vi "MosaicFocus.vi"() -> ()   [LabVIEW 2012]
uses:
  <vilib>/Utility/file.llb/Write To Spreadsheet File (DBL).vi
panel:
  in  "Track file":path
  in  "Piezo file":path=path "C:/Users/Ludovico/Lavoro/Experiments/Autofocus/vermi/CONFSTAGELOG/2016_12_16_10_06.txt"
  in  "Stage file":path=path "C:/Users/Ludovico/Lavoro/Experiments/Autofocus/vermi/CONFSTAGELOG/2016_12_16_10_06.txt"
  out "error out":errorcluster
  in  "error in (no error)":errorcluster
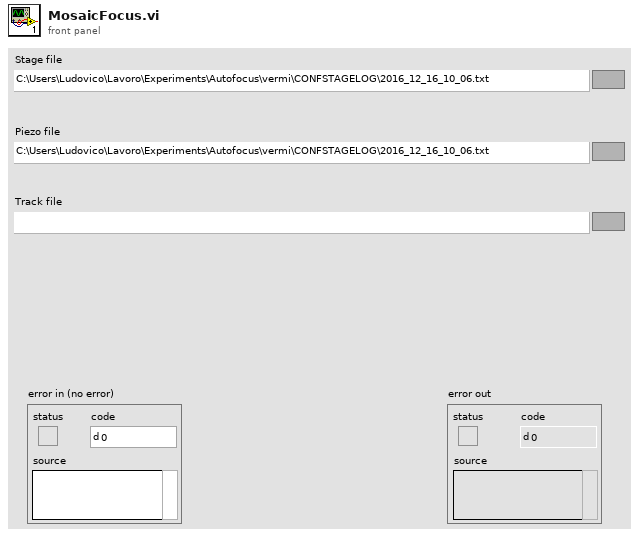
[diagram p1: front panel]
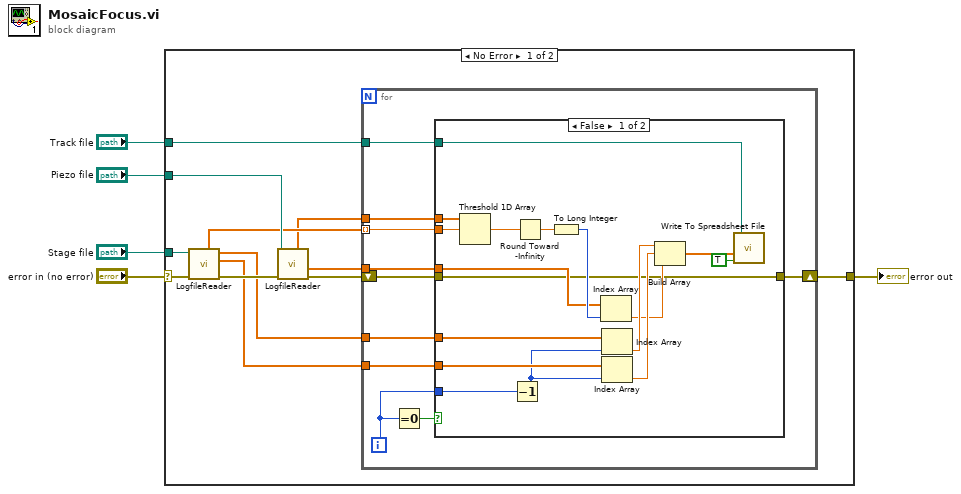
[diagram p0: block diagram]
diagram:
  n1 = case shown="No Error" "error in (no error)" {
    selector: "error in (no error)" -> [w17 w46]
    tunnel: [w6 w46] -> w4
    tunnel: "Stage file" -> [w16 _]
    tunnel: "Piezo file" -> [w14 _]
    tunnel: "Track file" -> [w8 _]
    frame No Error {
      n2 = call "LogfileReader.vi"("error in (no error)"=w17, "Positions file"=w16) -> ("error out"=w15:errorcluster, "Y"=w10:dbl[], "X"=w11:dbl[], "Time"=w13:dbl[])  [unwired: 5 in, 1 out]
      n3 = call "LogfileReader.vi"("error in (no error)"=w15, "Positions file"=w14) -> ("error out"=w7:errorcluster, "Focus"=w9:dbl[], "Time"=w12:dbl[])  [unwired: 5 in, 2 out]
      n4 = for {
        tunnel: w13 -> [w27] mode=indexing
        tunnel: w12 -> [w26]
        tunnel: w11 -> [w24]
        tunnel: w10 -> [w23]
        tunnel: w9 -> [w21]
        tunnel: w8 -> [w22]
        shift-right: [w19] -> w6
        shift-left: w7 -> [w20]
        i -> [w18]
        n5 = Equal To 0?(x=w18) -> (x = 0?=w25:bool)
        n6 = case shown="False" w25 {
          tunnel: w27 -> [w44 _]
          tunnel: w26 -> [w41 _]
          tunnel: w24 -> [w40 _]
          tunnel: w23 -> [w39 _]
          tunnel: w22 -> [w32 _]
          tunnel: w21 -> [w31 _]
          tunnel: w20 -> [w30 w45]
          tunnel: [w30 w45] -> w19
          tunnel: w18 -> [w29 _]
          frame False {
            n7 = Threshold 1D Array(2:w44, 3:w41) -> (0:w43:dbl)  [unwired: 1 in]
            n8 = Decrement(x=w29) -> (x-1=w28:i32)
            n9 = Round Toward -Infinity(1:w43) -> (0:w42:dbl)
            n10 = To Long Integer(number=w42) -> (32bit integer=w38:i32)
            n11 = Index Array(array=w31, index=w38) -> (element=w34:dbl)
            n12 = Index Array(array=w40, index=w28) -> (element=w36:dbl)
            n13 = Index Array(array=w39, index=w28) -> (element=w35:dbl)
            n14 = Build Array(w36, w35, w34) -> (w33:dbl[])
            n15 = call-poly <vilib>:"Write To Spreadsheet File.vi"("append to file? (new file:F)"=TRUE, "1D data"=w33, "file path (dialog if empty)"=w32) -> ()  [unwired: 5 in, 1 out]
          }
          frame True {
          }
        }
      }
    }
    frame Error {
    }
  }
  "error out" <- w4
